vi "get_command_by_name.vi"(8 "error in (no error)":errorcluster, 10 "name_to_search":string, 11 "Protocol_Generic in":refnum<class "Protocol_Generic.lvclass">) -> (0 "error out":errorcluster, 2 "command out":refnum<class "command_generic.lvclass">, 3 "Protocol_Generic out":refnum<class "Protocol_Generic.lvclass">)   [LabVIEW 2015, in "Protocol_Generic.lvclass"]
uses:
  Protocol_Generic.lvclass
  command/command_generic.lvclass
  Protocol_Generic.lvclass/Protocol_Generic.ctl
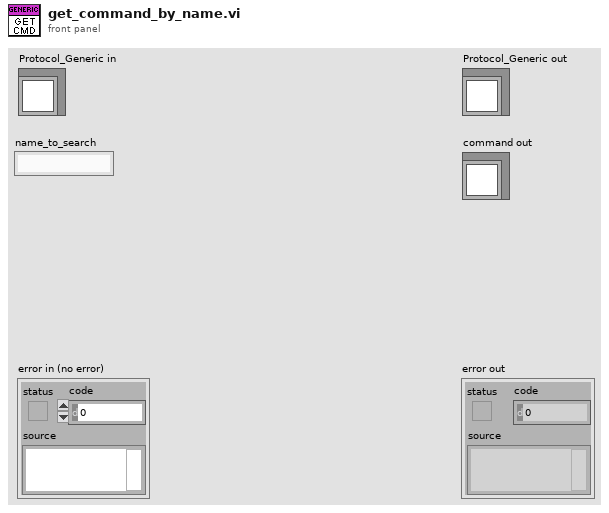
[diagram p1: front panel]
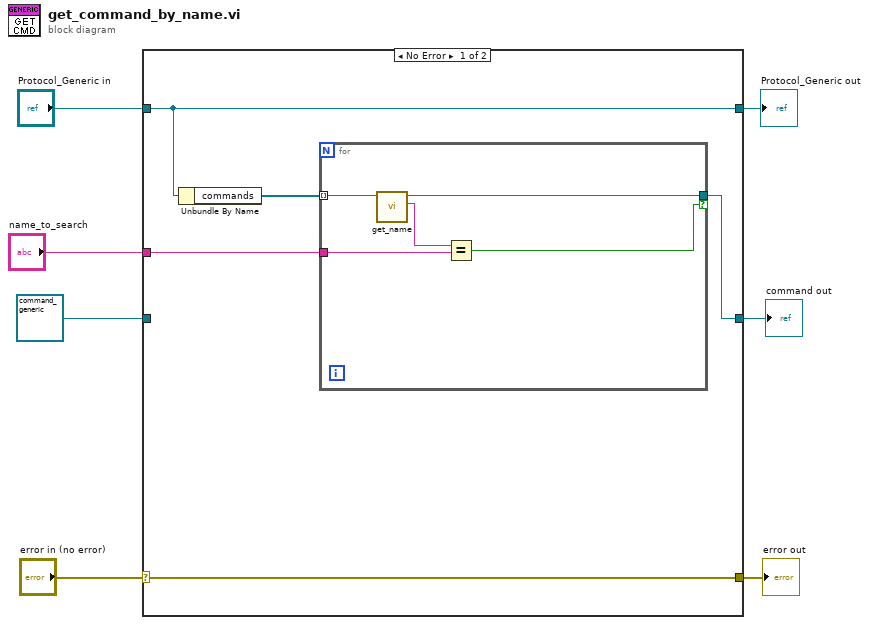
[diagram p0: block diagram]
diagram:
  n1 = case shown="No Error" "error in (no error)" {
    selector: "error in (no error)" -> [w12 w20]
    tunnel: [w12 w20] -> w6
    tunnel: [w11 w19] -> w4
    tunnel: "Protocol_Generic in" -> [w11 w19]
    tunnel: "name_to_search" -> [w9 _]
    tunnel: refnum<class "command_generic.lvclass"> refnum ("command_generic.lvclass") -> [_ w18]
    tunnel: [w8 w18] -> w1
    frame No Error {
      n2 = Unbundle By Name(w11) -> ("commands"=w10:refnum<class "command_generic.lvclass">[])
      n3 = for {
        tunnel: w10 -> [w17] mode=indexing
        tunnel: w9 -> [w15]
        tunnel: [w13] -> w8 if=w14
        n4 = call-dynamic "get_name.vi"("command in"=w17) -> ("name"=w16:string, "command out"=w13:refnum<class "command_generic.lvclass">)  [unwired: 8 in, 1 out]
        n5 = Equal?(x=w16, y=w15) -> (x = y?=w14:bool)
      }
    }
    frame Error {
    }
  }
  "error out" <- w6
  "Protocol_Generic out" <- w4
  "command out" <- w1
